vi "Img_Center_Crop.vi"(6 "Image Dst":T1, 8 "error in (no error)":errorcluster, 9 "height":i32, 10 "width":i32, 11 "Image In":T1) -> (0 "error out":errorcluster, 3 "Image Out":T1)   [LabVIEW 2020]
uses:
  <vilib>/vision/Image Controls.llb/IMAQ Image.ctl
  <vilib>/vision/NI_Vision_Development_Module.lvlib
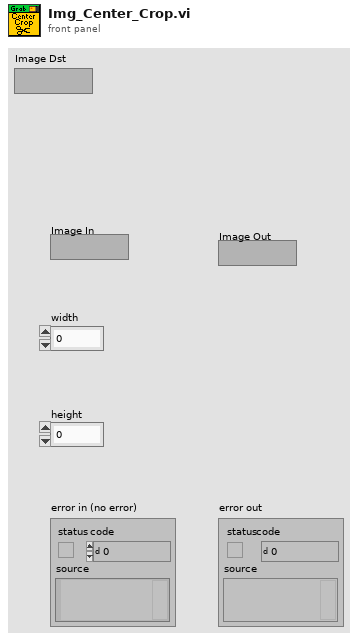
[diagram p1: front panel]
types:
  T1 = typedef "IMAQ Image.ctl" = refnum<image>
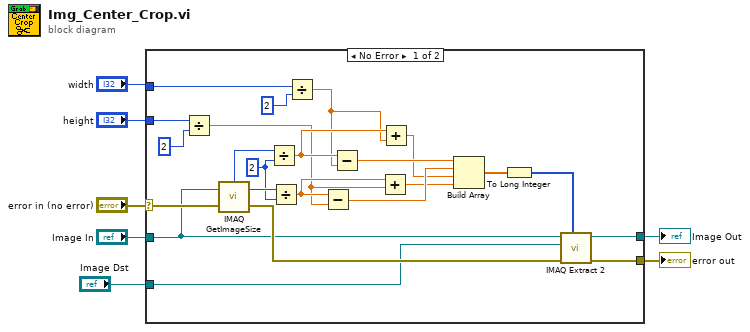
[diagram p0: block diagram]
diagram:
  n1 = case shown="No Error" "error in (no error)" {
    selector: "error in (no error)" -> [w11 w32]
    tunnel: "width" -> [w27 _]
    tunnel: "height" -> [w24 _]
    tunnel: [w14 w31] -> w5
    tunnel: "Image In" -> [w10 _]
    tunnel: [w9 w32] -> w2
    tunnel: "Image Dst" -> [w8 w31]
    frame No Error {
      w28 = 2
      n2 = Divide(x=w24, y=2) -> (x/y=w20:dbl)
      n3 = call "IMAQ GetImageSize"("Image"=w10, "error in (no error)"=w11) -> ("Y Resolution"=w30:i32, "X Resolution"=w29:i32, "error out"=w12:errorcluster)  [unwired: 2 in]
      n4 = Divide(x=w29, y=w28) -> (x/y=w23:dbl)
      n5 = Divide(x=w30, y=w28) -> (x/y=w21:dbl)
      n6 = Divide(x=w27, y=2) -> (x/y=w22:dbl)
      n7 = Subtract(x=w21, y=w20) -> (x-y=w18:dbl)
      n8 = Subtract(x=w23, y=w22) -> (x-y=w19:dbl)
      n9 = Add(x=w21, y=w20) -> (x+y=w16:dbl)
      n10 = Add(x=w23, y=w22) -> (x+y=w17:dbl)
      n11 = Build Array(w19, w18, w17, w16) -> (w15:dbl[])
      n12 = To Long Integer(number=w15) -> (32bit integer=w13:i32[])
      n13 = call "IMAQ Extract 2"("Optional Rectangle"=w13, "error in (no error)"=w12, "Image Dst"=w8, "Image Src"=w10) -> ("error out"=w9:errorcluster, "Image Dst Out"=w14:T1)  [unwired: 6 in]
    }
    frame Error {
    }
  }
  "Image Out" <- w5
  "error out" <- w2
